vi "ReadIntegerGlobals.vi"(8 "error in (no error)":errorcluster, 9 "variable count":i32, 10 "variable number":i32, 11 "controller in":refnum<k24>) -> (0 "error out":errorcluster, 2 "values":i32[](array[numeric]), 3 "controller out":refnum<k24>)   [LabVIEW 2010]
uses:
  c:/aerotech/controller/5.xx.xxx/ensemble/pc/labview/2010/bin/Aerotech.Ensemble.dll
  bin/Aerotech.Ensemble.dll
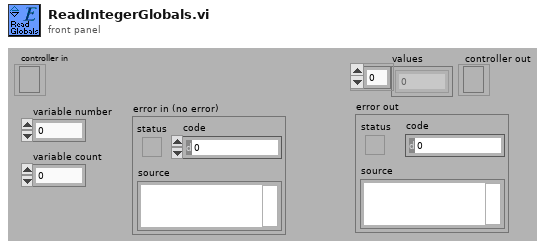
[diagram p1: front panel]
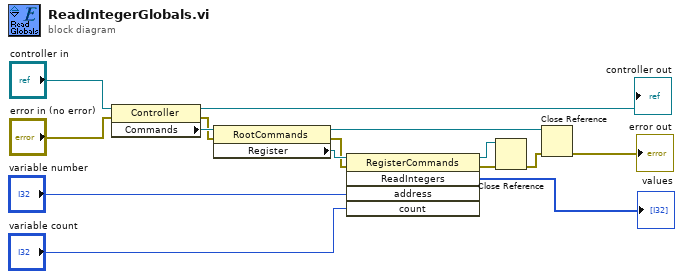
[diagram p0: block diagram]
diagram:
  n1 = property class="Controller"(reference="controller in", error in="error in (no error)") -> (reference out=→"controller out":refnum<k24>, error out=w4:errorcluster, "Commands"=w15:refnum<k24>)
  n2 = property class="RootCommands"(reference=w15, error in=w4) -> (reference out=w7:refnum<k24>, error out=w3:errorcluster, "Register"=w14:refnum<k24>)
  n3 = invoke class="RegisterCommands" method="ReadIntegers"(reference=w14, error in=w3, "address"="variable number", "count"="variable count") -> (reference out=w2:refnum<k24>, error out=w8:errorcluster, "ReadIntegers"=→"values":i32[])  [unwired: 1 in, 2 out]
  n4 = Close Reference(reference=w2, error in (no error)=w8) -> (error out=w1:errorcluster)
  n5 = Close Reference(reference=w7, error in (no error)=w1) -> (error out=→"error out":errorcluster)
